vi "Construct Ozone Step Sequence.vi"(8 "error in (no error)":errorcluster, 10 "QO2 DVR":refnum<data-value>, 11 "Seq Builder in":refnum<class "Cal Sequence Builder.lvclass">) -> (0 "error out":errorcluster, 2 "Steps":refnum<class "STEP.lvclass">[](array[class]), 3 "Seq Builder out":refnum<class "Cal Sequence Builder.lvclass">)   [LabVIEW 2015, in "Cal Sequence Builder.lvclass"]
uses:
  Cal Sequence Builder.lvclass
  Reusable/Sequence/STEPS/STEP.lvclass
  Set QO2 Rel Flow/Set Rel QO2 flow.lvclass
  Reusable/Data/Array Data/Single 1-D/Single_Array.lvclass
  config data.ctl
  Data/cPAS Data.lvclass
  Collect Data/Collect Data.lvclass
  Reusable/Data/U16/U16.lvclass
  Associated data/Associated Data.lvclass
  Data DVR/cPAS Data DVR.lvclass
  CRDS/Data/cCRDS Data.lvclass
  Wait/Wait.lvclass
  Reusable/Data/Double/Double.lvclass
  Reusable/Sequence/Sequence Factory/Sequence Builder.lvclass/Sequence Builder.ctl
  Cal Sequence Builder.lvclass/Cal Sequence Builder.ctl
  Wait/Wait.lvclass/Wait.ctl
  Data DVR/cPAS Data DVR.lvclass/cPAS Data DVR.ctl
  Associated data/Associated Data.lvclass/Associated Data.ctl
  Collect Data/Collect Data.lvclass/Collect Data.ctl
  Reusable/Sequence/STEPS/LEAVES/Double/Switch DBL.lvclass/Switch DBL.ctl
  Set QO2 Rel Flow/Set Rel QO2 flow.lvclass/Set Rel QO2 flow.ctl
  Reusable/Sequence/STEPS/LEAVES/Double/Write val.vi
  Set QO2 Rel Flow/Write QO2 DVR.vi
  Reusable/Sequence/Sequence Factory/Accessors/Read Config Data.vi
  Read Stored State DVR.vi
  Collect Data/Write PAS DVR.vi
  Collect Data/Write # of Obs.vi
  Collect Data/Write Associated Cells.vi
  Collect Data/Write Stored State DVR.vi
  Collect Data/Write CRD DVR.vi
  Reusable/Data/Data.lvclass
  State data/State Data.lvclass
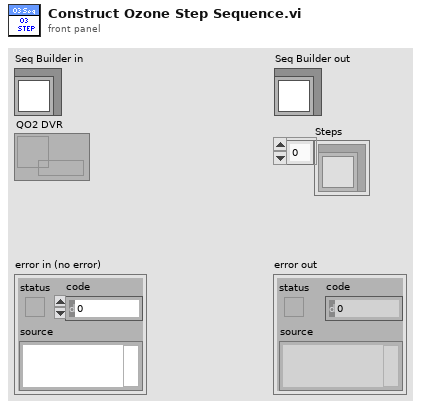
[diagram p1: front panel]
types:
  T1 = typedef "Cal Sequence Builder.lvclass/config data.ctl" = enum16{"purge time", "zero time", "qo2", "o3 stability", "laser stability", "pas state dvr", "collection observations", "associated cells", "crds state dvr", "Init Filter State"}
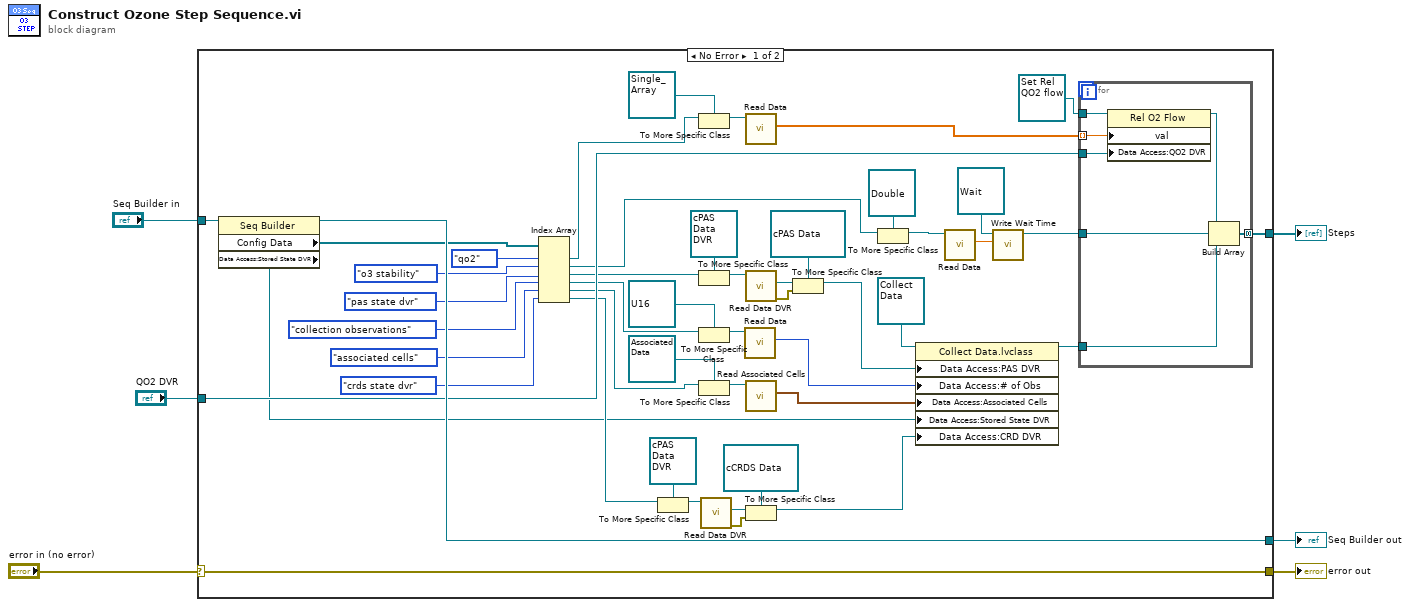
[diagram p0: block diagram]
diagram:
  n1 = case shown="No Error" "error in (no error)" {
    selector: "error in (no error)" -> [w54 w63]
    tunnel: [w54 w63] -> w5
    tunnel: [w48 w62] -> w3
    tunnel: "Seq Builder in" -> [w49 w62]
    tunnel: "QO2 DVR" -> [w44 _]
    tunnel: [w16 _] -> w1
    frame No Error {
      n2 = property class="Seq Builder"(reference=w49) -> (reference out=w48:refnum<class "Cal Sequence Builder.lvclass">, "Config Data"=w47:refnum<class "Data.lvclass">[], "Data Access:Stored State DVR"=w15:refnum<data-value>)  [unwired: 1 in, 1 out]
      n3 = Index Array(array=w47, index #1=config_data."qo2" ("config data"), index #2=config_data."o3 stability" ("config data"), index #3=config_data."pas state dvr" ("config data"), index #4=config_data."collection observations" ("config data"), index #5=config_data."associated cells" ("config data"), index #6=config_data."crds state dvr" ("config data")) -> (element #1=w45:refnum<class "Data.lvclass">, element #2=w10:refnum<class "Data.lvclass">, element #3=w37:refnum<class "Data.lvclass">, element #4=w30:refnum<class "Data.lvclass">, element #5=w26:refnum<class "Data.lvclass">, element #6=w18:refnum<class "Data.lvclass">)
      n4 = To More Specific Class(target class=refnum<class "cPAS Data DVR.lvclass"> refnum ("cPAS Data DVR.lvclass"), reference=w18) -> (specific class reference=w22:refnum<class "cPAS Data DVR.lvclass">)  [unwired: 1 in, 1 out]
      n5 = To More Specific Class(target class=refnum<class "Single_Array.lvclass"> refnum ("Base Data Class.lvlib:Single_Array.lvclass"), reference=w45) -> (specific class reference=w51:refnum<class "Single_Array.lvclass">)  [unwired: 1 in, 1 out]
      n6 = To More Specific Class(target class=refnum<class "cPAS Data DVR.lvclass"> refnum ("cPAS Data DVR.lvclass"), reference=w37) -> (specific class reference=w40:refnum<class "cPAS Data DVR.lvclass">)  [unwired: 1 in, 1 out]
      n7 = To More Specific Class(target class=refnum<class "U16.lvclass"> refnum ("Base Data Class.lvlib:U16"), reference=w30) -> (specific class reference=w32:refnum<class "U16.lvclass">)  [unwired: 1 in, 1 out]
      n8 = To More Specific Class(target class=refnum<class "Associated Data.lvclass"> refnum ("Associated Data.lvclass"), reference=w26) -> (specific class reference=w27:refnum<class "Associated Data.lvclass">)  [unwired: 1 in, 1 out]
      n9 = call "Read Data DVR.vi"("cPAS Data DVR in"=w22) -> ("error out"=w21:errorcluster, "Data DVR"=w20:refnum<data-value>)  [unwired: 8 in, 1 out]
      n10 = call "Read Data.vi"("U16 in"=w32) -> ("Data"=w8:u16)  [unwired: 8 in, 2 out]
      n11 = call "Read Data.vi"("Single_Array in"=w51) -> ("Data"=w50:sgl[])  [unwired: 8 in, 2 out]
      n12 = call "Read Data DVR.vi"("cPAS Data DVR in"=w40) -> ("error out"=w39:errorcluster, "Data DVR"=w38:refnum<data-value>)  [unwired: 8 in, 1 out]
      n13 = call "Read Associated Cells.vi"("Associated Data in"=w27) -> ("Associated Cells"=w25:cluster{"PAS":dbl, "CRD":dbl}[])  [unwired: 8 in, 2 out]
      n14 = To More Specific Class(target class=refnum<data-value> refnum ("Data DVR"), reference=w20, error in=w21) -> (specific class reference=w17:refnum<data-value>)  [unwired: 1 out]
      n15 = To More Specific Class(target class=refnum<data-value> refnum ("Data DVR"), reference=w38, error in=w39) -> (specific class reference=w7:refnum<data-value>)  [unwired: 1 out]
      n16 = To More Specific Class(target class=refnum<class "Double.lvclass"> refnum ("Base Data Class.lvlib:Double.lvclass"), reference=w10) -> (specific class reference=w11:refnum<class "Double.lvclass">)  [unwired: 1 in, 1 out]
      n17 = property class="Collect Data.lvclass"(reference=refnum<class "Collect Data.lvclass"> refnum ("Collect Data.lvclass"), "Data Access:PAS DVR"=w7, "Data Access:# of Obs"=w8, "Data Access:Associated Cells"=w25, "Data Access:Stored State DVR"=w15, "Data Access:CRD DVR"=w17) -> (reference out=w34:refnum<class "Collect Data.lvclass">)  [unwired: 1 in, 1 out]
      n18 = call "Read Data.vi"("Double in"=w11) -> ("Data"=w12:dbl)  [unwired: 8 in, 2 out]
      n19 = call "Write Wait Time.vi"("Wait Time"=w12, "Wait in"=refnum<class "Wait.lvclass"> refnum ("Wait")) -> ("Wait out"=w9:refnum<class "Wait.lvclass">)  [unwired: 8 in, 1 out]
      n20 = for {
        tunnel: w50 -> [w60] mode=indexing
        tunnel: refnum<class "Set Rel QO2 flow.lvclass"> refnum ("Rel O2 Flow") -> [w61]
        tunnel: w44 -> [w59]
        tunnel: w9 -> [w57]
        tunnel: [w56] -> w16 mode=concatenating
        tunnel: w34 -> [w55]
        n21 = property class="Rel O2 Flow"(reference=w61, "val"=w60, "Data Access:QO2 DVR"=w59) -> (reference out=w58:refnum<class "Set Rel QO2 flow.lvclass">)  [unwired: 1 in, 1 out]
        n22 = Build Array(w58, w57, w55) -> (w56:refnum<class "STEP.lvclass">[])
      }
    }
    frame Error {
    }
  }
  "error out" <- w5
  "Seq Builder out" <- w3
  "Steps" <- w1
